vi "AWG Stop Pulses.vi"(8 "error in (no error)":errorcluster, 11 "awg session in":T1={"type"=enum."Agilent 331xxA to 332xxA", "VISA"="", "enable 10MHz ref"=FALSE, "cmi ckd2"={"VISA"="", "clock source"=enum."Auto", "manual ref clk"=FALSE, "ref clock [Hz]"=0.0, "div mode"=enum."Set divisor directly"}, "cmi sync v3"={"VISA"="", "baud rate [bd/s]"=115200, "source"=enum."Auto", "hv range"=enum."1kV", "fsrc is fixed"=FALSE, "fsrc [Hz]"=10000000.0, "freq integ [s]"=1.0, "freq filter"=5, "trig level"=enum."TTL 5V", "chn1 mode"=enum."Source divider", "chn1 level"=enum."Positive 5V", "chn2 mode"=enum."Source divider", "chn2 level"=enum."Positive 5V", "chn2 div"=1, "chn3 mode"=enum."Chn 1 Active", "chn3 level"=enum."Positive 5V", "chn1 div entry"=enum."Calculate nearest divisor from measured fx", "chn1 dev limit [%]"=1.0, "chn1 check dev"=FALSE}, "trigger"={"source"=enum."Immediate", "level [V]"=0.0, "coupling"=enum."DC", "slope"=enum."POS"}, "HMF2500 cfg"={"Baud Rate"=9600, "Parity"=0, "Data Bits"=8, "Flow Control"=4}} {"HMF2500 cfg"."Flow Control" items=["None", "XON/XOFF", "RTS/CTS", "XON/XOFF & RTS/CTS", "DTR/DSR", "XON/XOFF & DTR/DSR"]; "HMF2500 cfg"."Data Bits" items=["7"=7, "8"=8]; "HMF2500 cfg"."Parity" items=["None", "Odd", "Even", "Mark", "Space"]; "HMF2500 cfg"."Baud Rate" items=["300"=300, "600"=600, "1200"=1200, "2400"=2400, "4800"=4800, "9600"=9600, "19200"=19200]; "cmi sync v3"."chn2 div" min=1 max=100000000 step=1; "cmi sync v3"."fsrc [Hz]" format="%_8p"}) -> (0 "error out":errorcluster, 3 "awg session out":T1={"type"=enum."Agilent 331xxA to 332xxA", "VISA"="", "enable 10MHz ref"=FALSE, "cmi ckd2"={"VISA"="", "clock source"=enum."Auto", "manual ref clk"=FALSE, "ref clock [Hz]"=0.0, "div mode"=enum."Set divisor directly"}, "cmi sync v3"={"VISA"="", "baud rate [bd/s]"=115200, "source"=enum."Auto", "hv range"=enum."1kV", "fsrc is fixed"=FALSE, "fsrc [Hz]"=10000000.0, "freq integ [s]"=1.0, "freq filter"=5, "trig level"=enum."TTL 5V", "chn1 mode"=enum."Source divider", "chn1 level"=enum."Positive 5V", "chn2 mode"=enum."Source divider", "chn2 level"=enum."Positive 5V", "chn2 div"=1, "chn3 mode"=enum."Chn 1 Active", "chn3 level"=enum."Positive 5V", "chn1 div entry"=enum."Calculate nearest divisor from measured fx", "chn1 dev limit [%]"=1.0, "chn1 check dev"=FALSE}, "trigger"={"source"=enum."Immediate", "level [V]"=0.0, "coupling"=enum."DC", "slope"=enum."POS"}, "HMF2500 cfg"={"Baud Rate"=9600, "Parity"=0, "Data Bits"=8, "Flow Control"=4}} {"HMF2500 cfg"."Flow Control" items=["None", "XON/XOFF", "RTS/CTS", "XON/XOFF & RTS/CTS", "DTR/DSR", "XON/XOFF & DTR/DSR"]; "HMF2500 cfg"."Data Bits" items=["7"=7, "8"=8]; "HMF2500 cfg"."Parity" items=["None", "Odd", "Even", "Mark", "Space"]; "HMF2500 cfg"."Baud Rate" items=["300"=300, "600"=600, "1200"=1200, "2400"=2400, "4800"=4800, "9600"=9600, "19200"=19200]; "cmi sync v3"."chn2 div" min=1 max=100000000 step=1; "cmi sync v3"."fsrc [Hz]" format="%_8p"})   [LabVIEW 2020, in "AWG.lvlib"]
doc: "AWG wrapper: Stops generation of pulses at output. At least for 33120 model this should be called first after initialization to stop standard waveform mode, i.e. to stop output."
uses:
  AWG.lvlib
  Agilent 33XXX Series/Agilent 33XXX Series.lvlib
  AFG3000/Tektronix AFG 3000 Series.lvlib
  CMI Sync V3/CMI Sync Unit V3.lvlib
  CMI Sync V3/Configure/CMI Sync V3 Trigger Mode.ctl
  AWG Type.ctl
  AWG Session.ctl
  CMI Clock Divider v2/CMI ckd2 Source Mode.ctl
  CMI Clock Divider v2/CMI ckd2 Session.ctl
  CMI Sync V3/Configure/CMI Sync V3 Reference Clock Source.ctl
  CMI Sync V3/Configure/CMI Sync V3 HV input Range.ctl
  CMI Sync V3/Configure/CMI Sync V3 Trigger Input Level.ctl
  CMI Sync V3/Configure/CMI Sync V3 Channel 1 Mode.ctl
  CMI Sync V3/Configure/CMI Sync V3 Channel Output Levels.ctl
  CMI Sync V3/Configure/CMI Sync V3 Channel 2 Mode.ctl
  CMI Sync V3/Configure/CMI Sync V3 Channel 3 Mode.ctl
  CMI Sync V3/CMI Sync V3 session.ctl
  externals needed for AWG/ADC Trig Mode Source.ctl
  externals needed for AWG/ADC Trig Coupling.ctl
  externals needed for AWG/ADC Trig Slope.ctl
  externals needed for AWG/ADC Trig Config.ctl
  CMI Sync V3/Configure/CMI Sync V3 Channel 1 Divisor Entry Mode.ctl
  CMI Clock Divider v2/CMI ckd2 Divisor Mode.ctl
  RaS HMF2500/HMF2500 Config.ctl
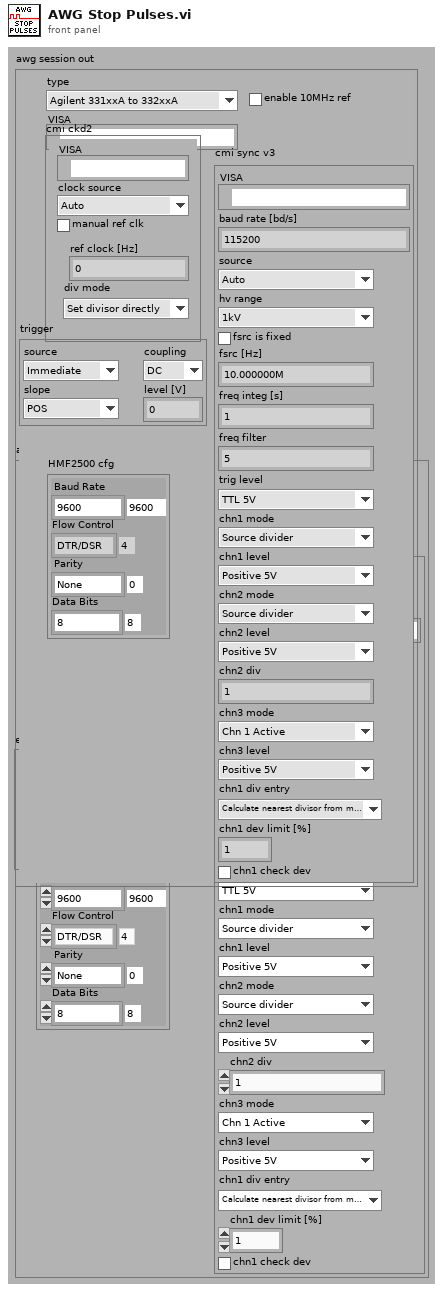
[diagram p1: front panel]
types:
  T1 = typedef "AWG.lvlib/AWG Session.ctl" = cluster{"type":T2, "VISA":refnum<visa-resource-name>, "enable 10MHz ref":bool, "cmi ckd2":T3, "cmi sync v3":T6, "trigger":T15, "HMF2500 cfg":T19}
  T2 = typedef "AWG.lvlib/AWG Type.ctl" = enum16{"Agilent 331xxA to 332xxA", "Agilent 335xxA to 336xxA", "Tektronix AFG3101C", "R&S HMF25xx", "CMI Clock Divider v2", "CMI Sync Unit V3", "dummy"}
  T3 = typedef "AWG.lvlib/CMI ckd2 Session.ctl" = cluster{"VISA":refnum<visa-resource-name>, "clock source":T4, "manual ref clk":bool, "ref clock [Hz]":dbl, "div mode":T5}
  T4 = typedef "AWG.lvlib/CMI ckd2 Source Mode.ctl" = enum16{"Auto", "LF clock", "HF clock", "Internal"}
  T5 = typedef "AWG.lvlib/CMI ckd2 Divisor Mode.ctl" = enum16{"Set divisor directly", "Set divisor by frequency"}
  T6 = typedef "AWG.lvlib/CMI Sync Unit V3.lvlib/CMI Sync V3 session.ctl" = cluster{"VISA":refnum<visa-resource-name>, "baud rate [bd/s]":i32, "source":T7, "hv range":T8, "fsrc is fixed":bool, "fsrc [Hz]":dbl, "freq integ [s]":dbl, "freq filter":i32, "trig level":T9, "chn1 mode":T10, "chn1 level":T11, "chn2 mode":T12, "chn2 level":T11, "chn2 div":i32, "chn3 mode":T13, "chn3 level":T11, "chn1 div entry":T14, "chn1 dev limit [%]":dbl, "chn1 check dev":bool}
  T7 = typedef "AWG.lvlib/CMI Sync Unit V3.lvlib/CMI Sync V3 Reference Clock Source.ctl" = enum16{"Auto", "Internal", "Logic", "Sine", "HV"}
  T8 = typedef "AWG.lvlib/CMI Sync Unit V3.lvlib/CMI Sync V3 HV input Range.ctl" = enum16{"10V", "60V", "250V", "1kV"}
  T9 = typedef "AWG.lvlib/CMI Sync Unit V3.lvlib/CMI Sync V3 Trigger Input Level.ctl" = enum16{"LVCMOS 3V3", "TTL 5V"}
  T10 = typedef "AWG.lvlib/CMI Sync Unit V3.lvlib/CMI Sync V3 Channel 1 Mode.ctl" = enum16{"Source divider", "DDS absolute", "DDS ratio", "DDS ratio M/N"}
  T11 = typedef "AWG.lvlib/CMI Sync Unit V3.lvlib/CMI Sync V3 Channel Output Levels.ctl" = enum16{"Positive 3V3", "Negative 3V3", "Positive 5V", "Negative 5V"}
  T12 = typedef "AWG.lvlib/CMI Sync Unit V3.lvlib/CMI Sync V3 Channel 2 Mode.ctl" = enum16{"Source divider", "Chn 1 divide"}
  T13 = typedef "AWG.lvlib/CMI Sync Unit V3.lvlib/CMI Sync V3 Channel 3 Mode.ctl" = enum16{"Chn 1 Active", "Chn 2 Active", "Chn 1 Trigger", "Chn 2 Trigger", "Gate", "PPS", "10MHz"}
  T14 = typedef "AWG.lvlib/CMI Sync Unit V3.lvlib/CMI Sync V3 Channel 1 Divisor Entry Mode.ctl" = enum16{"Set divisor directly", "Calculate nearest divisor from measured fx"}
  T15 = typedef "ADC Trig Config.ctl" = cluster{"source":T16, "level [V]":dbl, "coupling":T17, "slope":T18}
  T16 = typedef "ADC Trig Mode Source.ctl" = enum16{"Immediate", "External", "Level"}
  T17 = typedef "ADC Trig Coupling.ctl" = enum16{"DC", "AC"}
  T18 = typedef "ADC Trig Slope.ctl" = enum16{"POS", "NEG"}
  T19 = typedef "AWG.lvlib/HMF2500 Config.ctl" = cluster{"Baud Rate":u32, "Parity":u16, "Data Bits":u16, "Flow Control":u16}
  T20 = typedef "AWG.lvlib/CMI Sync Unit V3.lvlib/CMI Sync V3 Trigger Mode.ctl" = enum16{"Hold", "Auto (continuous)", "Gate positive", "Gate negative", "Rising edge", "Falling edge", "Bus (*TRG)", "Manual (button)"}
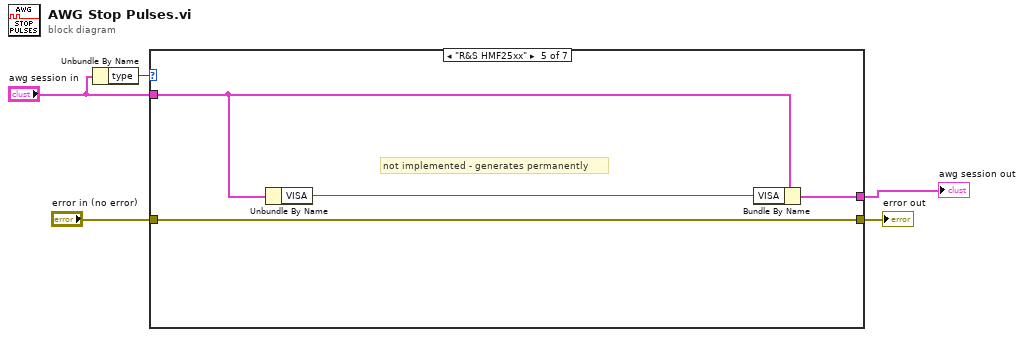
[diagram p0: block diagram]
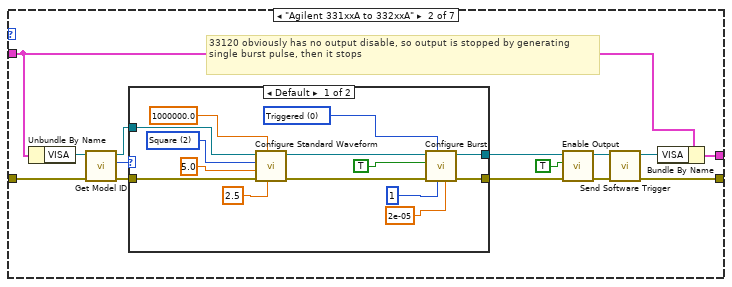
[diagram p3: hidden frame]
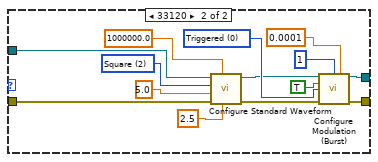
[diagram p4: hidden frame]
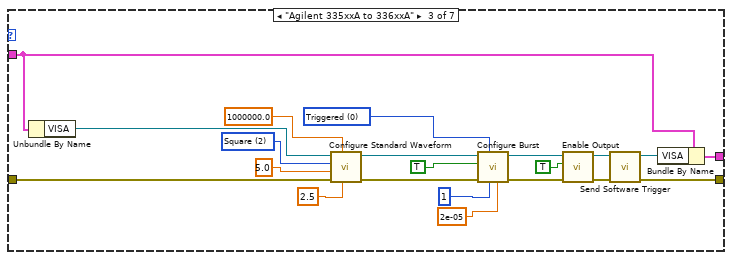
[diagram p5: hidden frame]
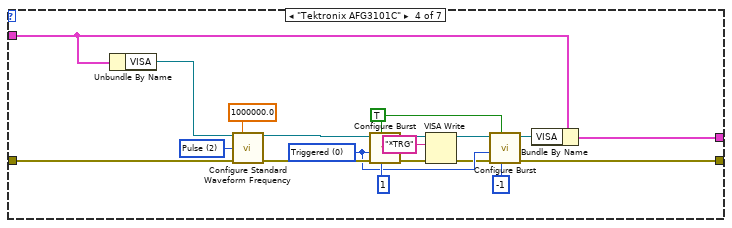
[diagram p6: hidden frame]
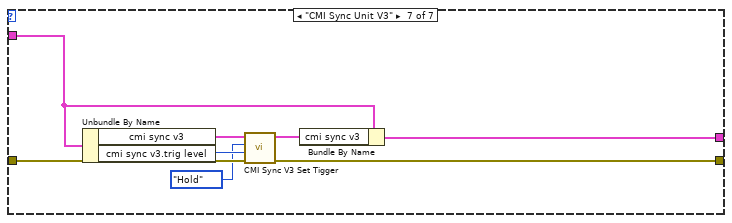
[diagram p8: hidden frame]
diagram:
  n1 = Unbundle By Name("awg session in") -> ("type"=w5:T2)
  n2 = case shown="\"R&S HMF25xx\"" w5 {
    tunnel: "error in (no error)" -> [w7 w19 w50 w86 w90 w95 w103]
    tunnel: [w7 w8 w62 w76 w90 w95 w99] -> w3
    tunnel: "awg session in" -> [w6 w20 w70 w88 w93 w94 w98]
    tunnel: [w6 w21 w69 w87 w91 w94 w96] -> w1
    frame Default {
    }
    frame "Agilent 331xxA to 332xxA" {
      # "33120 obviously has no output disable, so output is stopped by generating\nsingle burst pulse, then it stops"
      n3 = Unbundle By Name(w20) -> ("VISA"=w18:refnum<visa-resource-name>)
      n4 = call "Get Model ID.vi"("error in (no error)"=w19, "VISA resource name"=w18) -> ("error out"=w17:errorcluster, "model ID"=w15:u32, "VISA resource name out"=w16:refnum<visa-resource-name>)  [unwired: 7 in]
      n5 = case shown="Default" w15 {
        tunnel: [w31 w45] -> w13
        tunnel: [w30 w44] -> w12
        tunnel: w17 -> [w25 w43]
        tunnel: w16 -> [w24 w42]
        frame Default {
          w27 = u16 2 items=["DC", "Sine", "Square", "Triangle", "Ramp", "Pulse", "Noise", "Sinc", "Negative Ramp", "Exponential Rise", "Exponential Fall", "Cardiac"] ("Waveform Function (1: Sine)")
          w35 = u16 0 items=["Triggered", "Gated"] ("Burst Mode (0: Triggered)")
          n6 = call "Configure Standard Waveform.vi"("DC Offset (0.00 V)"=2.5, "Frequency (1000 Hz)"=1000000.0, "error in (no error)"=w25, "Amplitude (1)"=5.0, "Waveform Function (1: Sine)"=w27, "VISA resource name"=w24) -> ("error out"=w23:errorcluster, "VISA resource name out"=w22:refnum<visa-resource-name>)  [unwired: 4 in]
          n7 = call "Configure Burst.vi"("Burst Period (1 s)"=2e-05, "Burst Count (1)"=1, "Burst Mode (0: Triggered)"=w35, "error in (no error)"=w23, "Enable Burst (T: Enable)"=TRUE, "VISA resource name"=w22) -> ("error out"=w31:errorcluster, "VISA resource name out"=w30:refnum<visa-resource-name>)  [unwired: 4 in]
        }
        frame 33120 {
          w38 = u16 2 items=["DC", "Sine", "Square", "Triangle", "Ramp", "Pulse", "Noise", "Sinc", "Negative Ramp", "Exponential Rise", "Exponential Fall", "Cardiac"] ("Waveform Function (1: Sine)")
          w46 = u16 0 items=["Triggered", "Gated"] ("Burst Modulation Mode (0: Triggered)")
          n8 = call "Configure Standard Waveform.vi"("DC Offset (0.00 V)"=2.5, "Frequency (1000 Hz)"=1000000.0, "error in (no error)"=w43, "Amplitude (1)"=5.0, "Waveform Function (1: Sine)"=w38, "VISA resource name"=w42) -> ("error out"=w41:errorcluster, "VISA resource name out"=w40:refnum<visa-resource-name>)  [unwired: 4 in]
          n9 = call "Configure Modulation (Burst).vi"("VISA resource name"=w40, "Burst Count (1)"=1, "Burst Period (1 s)"=0.0001, "Enable Burst Modulation (T: Enable)"=TRUE, "Burst Modulation Mode (0: Triggered)"=w46, "error in (no error)"=w41) -> ("VISA resource name out"=w44:refnum<visa-resource-name>, "error out"=w45:errorcluster)  [unwired: 8 in]
        }
      }
      n10 = call "Enable Output.vi"("error in (no error)"=w13, "Enable Output  (T: Enable)"=TRUE, "VISA resource name"=w12) -> ("error out"=w11:errorcluster, "VISA resource name out"=w10:refnum<visa-resource-name>)  [unwired: 7 in]
      n11 = call "Send Software Trigger.vi"("error in (no error)"=w11, "VISA resource name"=w10) -> ("error out"=w8:errorcluster, "VISA resource name out"=w9:refnum<visa-resource-name>)  [unwired: 8 in]
      n12 = Bundle By Name(cluster=w20, "VISA"=w9) -> (w21:T1)
    }
    frame "Agilent 335xxA to 336xxA" {
      w55 = u16 2 items=["DC", "Sine", "Square", "Triangle", "Ramp", "Pulse", "Noise", "Sinc", "Negative Ramp", "Exponential Rise", "Exponential Fall", "Cardiac"] ("Waveform Function (1: Sine)")
      w61 = u16 0 items=["Triggered", "Gated"] ("Burst Mode (0: Triggered)")
      n13 = Unbundle By Name(w70) -> ("VISA"=w51:refnum<visa-resource-name>)
      n14 = call "Configure Standard Waveform.vi"("DC Offset (0.00 V)"=2.5, "Frequency (1000 Hz)"=1000000.0, "error in (no error)"=w50, "Amplitude (1)"=5.0, "Waveform Function (1: Sine)"=w55, "VISA resource name"=w51) -> ("error out"=w53:errorcluster, "VISA resource name out"=w52:refnum<visa-resource-name>)  [unwired: 4 in]
      n15 = call "Configure Burst.vi"("Burst Period (1 s)"=2e-05, "Burst Count (1)"=1, "Burst Mode (0: Triggered)"=w61, "error in (no error)"=w53, "Enable Burst (T: Enable)"=TRUE, "VISA resource name"=w52) -> ("error out"=w67:errorcluster, "VISA resource name out"=w66:refnum<visa-resource-name>)  [unwired: 4 in]
      n16 = call "Enable Output.vi"("error in (no error)"=w67, "Enable Output  (T: Enable)"=TRUE, "VISA resource name"=w66) -> ("error out"=w65:errorcluster, "VISA resource name out"=w64:refnum<visa-resource-name>)  [unwired: 7 in]
      n17 = call "Send Software Trigger.vi"("error in (no error)"=w65, "VISA resource name"=w64) -> ("error out"=w62:errorcluster, "VISA resource name out"=w63:refnum<visa-resource-name>)  [unwired: 8 in]
      n18 = Bundle By Name(cluster=w70, "VISA"=w63) -> (w69:T1)
    }
    frame "Tektronix AFG3101C" {
      w81 = u16 2 items=["Sine", "Square", "Pulse", "Ramp", "Noise", "DC", "Sin(x)/x", "Gaussian", "Lorentz", "Exponential Rise", "Exponential Decay", "Haversine"] ("Waveform Function (0: Sine)")
      w79 = TRUE ("Enable Burst (T: Enable)")
      w78 = u16 0 items=["Triggered", "Gated"] ("Burst Mode (0: Triggered)")
      n19 = Unbundle By Name(w88) -> ("VISA"=w83:refnum<visa-resource-name>)
      n20 = call "Configure Standard Waveform Frequency.vi"("VISA resource name"=w83, "Frequency (1000 Hz)"=1000000.0, "Waveform Function (0: Sine)"=w81, "error in (no error)"=w86) -> ("VISA resource name out"=w84:refnum<visa-resource-name>, "error out"=w85:errorcluster)  [unwired: 10 in]
      n21 = call "Configure Burst.vi"("Burst Count (5)"=1, "Enable Burst (T: Enable)"=w79, "error in (no error)"=w85, "Burst Mode (0: Triggered)"=w78, "VISA resource name"=w84) -> ("error out"=w75:errorcluster, "VISA resource name out"=w74:refnum<visa-resource-name>)  [unwired: 5 in]
      n22 = VISA Write(VISA resource name=w74, write buffer="*TRG", error in (no error)=w75) -> (VISA resource name out=w73:refnum<visa-resource-name>, error out=w72:errorcluster)  [unwired: 1 out]
      n23 = call "Configure Burst.vi"("Burst Count (5)"=-1, "Enable Burst (T: Enable)"=w79, "error in (no error)"=w72, "Burst Mode (0: Triggered)"=w78, "VISA resource name"=w73) -> ("error out"=w76:errorcluster, "VISA resource name out"=w77:refnum<visa-resource-name>)  [unwired: 5 in]
      n24 = Bundle By Name(cluster=w88, "VISA"=w77) -> (w87:T1)
    }
    frame "R&S HMF25xx" {
      # "not implemented - generates permanently"
      n25 = Unbundle By Name(w93) -> ("VISA"=w92:refnum<visa-resource-name>)
      n26 = Bundle By Name(cluster=w93, "VISA"=w92) -> (w91:T1)
    }
    frame "CMI Clock Divider v2" {
      # "not implemented - generates pulses continuously"
    }
    frame "CMI Sync Unit V3" {
      n27 = Unbundle By Name(w98) -> ("cmi sync v3"=w102:T6, "cmi sync v3.trig level"=w101:T9)
      n28 = call "CMI Sync V3 Set Tigger.vi"("error in"=w103, "Trigger input logic (5V)"=w101, "Trigger mode (Auto)"=CMI_Sync_V3_Trigger_Mode."Hold", "session in"=w102) -> ("error out"=w99:errorcluster, "session out"=w97:T6)  [unwired: 6 in]
      n29 = Bundle By Name(cluster=w98, "cmi sync v3"=w97) -> (w96:T1)
    }
  }
  "error out" <- w3
  "awg session out" <- w1
